vi "test-30frame-QR-static.vi"() -> ()   [LabVIEW 2015]
uses:
  <vilib>/MakerHub/LINX/Public/Peripherals/Digital/Digital Read 1 Chan.vi
  <vilib>/MakerHub/LINX/Public/Peripherals/Digital/Digital Read N Chans.vi
  <vilib>/MakerHub/LINX/Private/Local IO/LinxDigitalRead.vi
  <vilib>/MakerHub/LINX/Public/Utilities/Check Channel.vi
  <vilib>/MakerHub/LINX/Public/Utilities/Open Serial.vi
  <vilib>/MakerHub/LINX/Private/Utilties/Generate Error.vi
  <vilib>/MakerHub/LINX/LMH-LINX.lvlib
  <vilib>/gmath/NI_Gmath.lvlib
panel:
  in  "sensor pin":u8
  in  "Frequency (Hz)":u32=1600
  in  "DIR pin":u8=3
  in  "Pulse pin":u8=4
  out "Form code":bool
  in  "Sensor  Port":refnum<visa-resource-name>="COM3"
  out "data current = data previous ?":bool
  in  "Port Motor":refnum<visa-resource-name>="COM18"
  out "?":T1(plugin-control)
  in  "stop":bool
  out "data-global":string
  out "sum package":dbl
  out "Found?":bool
  out "Mass (kg):":dbl
  out "Tong K/lg (kg)":dbl
  out "Quantity":i32=50
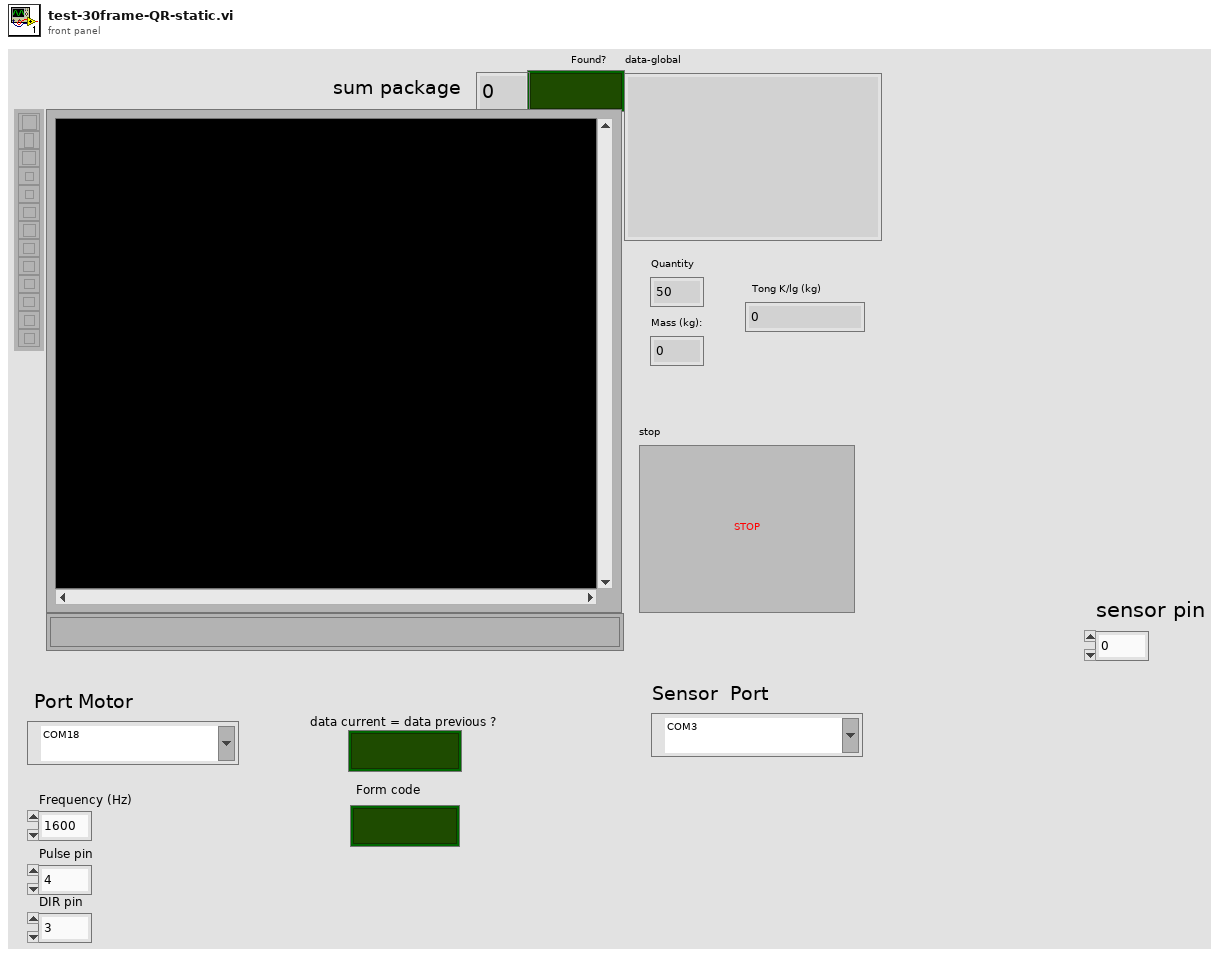
[diagram p1: front panel]
types:
  T1 = typedef "IMAQ Image.ctl" = refnum<image>
  T2 = typedef "LMH-LINX.lvlib/LINX Ref.ctl" = cluster{"IO":T3, "Interface":T4, "LINX Device Config":T5}
  T3 = typedef "LMH-LINX.lvlib/Platform.ctl" = enum16{"Remote", "Local"}
  T4 = typedef "LMH-LINX.lvlib/Interface.ctl" = enum16{"Serial", "TCP"}
  T5 = typedef "LMH-LINX.lvlib/Device.lvlib/LINX Device Config.ctl" = cluster{"Interface":T4, "COM Port":refnum<visa-resource-name>, "TCP Configuration":T6, "Device Family":u8, "Device ID":u8, "Device Name":string, "TCP Ref":refnum<k5>, "Channels":T7}
  T6 = typedef "LMH-LINX.lvlib/Device.lvlib/TCP Config.ctl" = cluster{"IP Address":string, "Port":u16}
  T7 = typedef "LMH-LINX.lvlib/Channels.ctl" = cluster{"DI":u8[], "DO":u8[], "AI":u8[], "AO":u8[], "PWM":u8[], "QE":u8[], "UART":u8[], "I2C 2":u8[], "SPI":u8[], "CAN":u8[], "Servo":u8[], "AI Ref (V)":dbl, "AI Resolution (Bits)":u8, "AO Ref (V)":dbl, "AO Resolution (Bits)":u8}
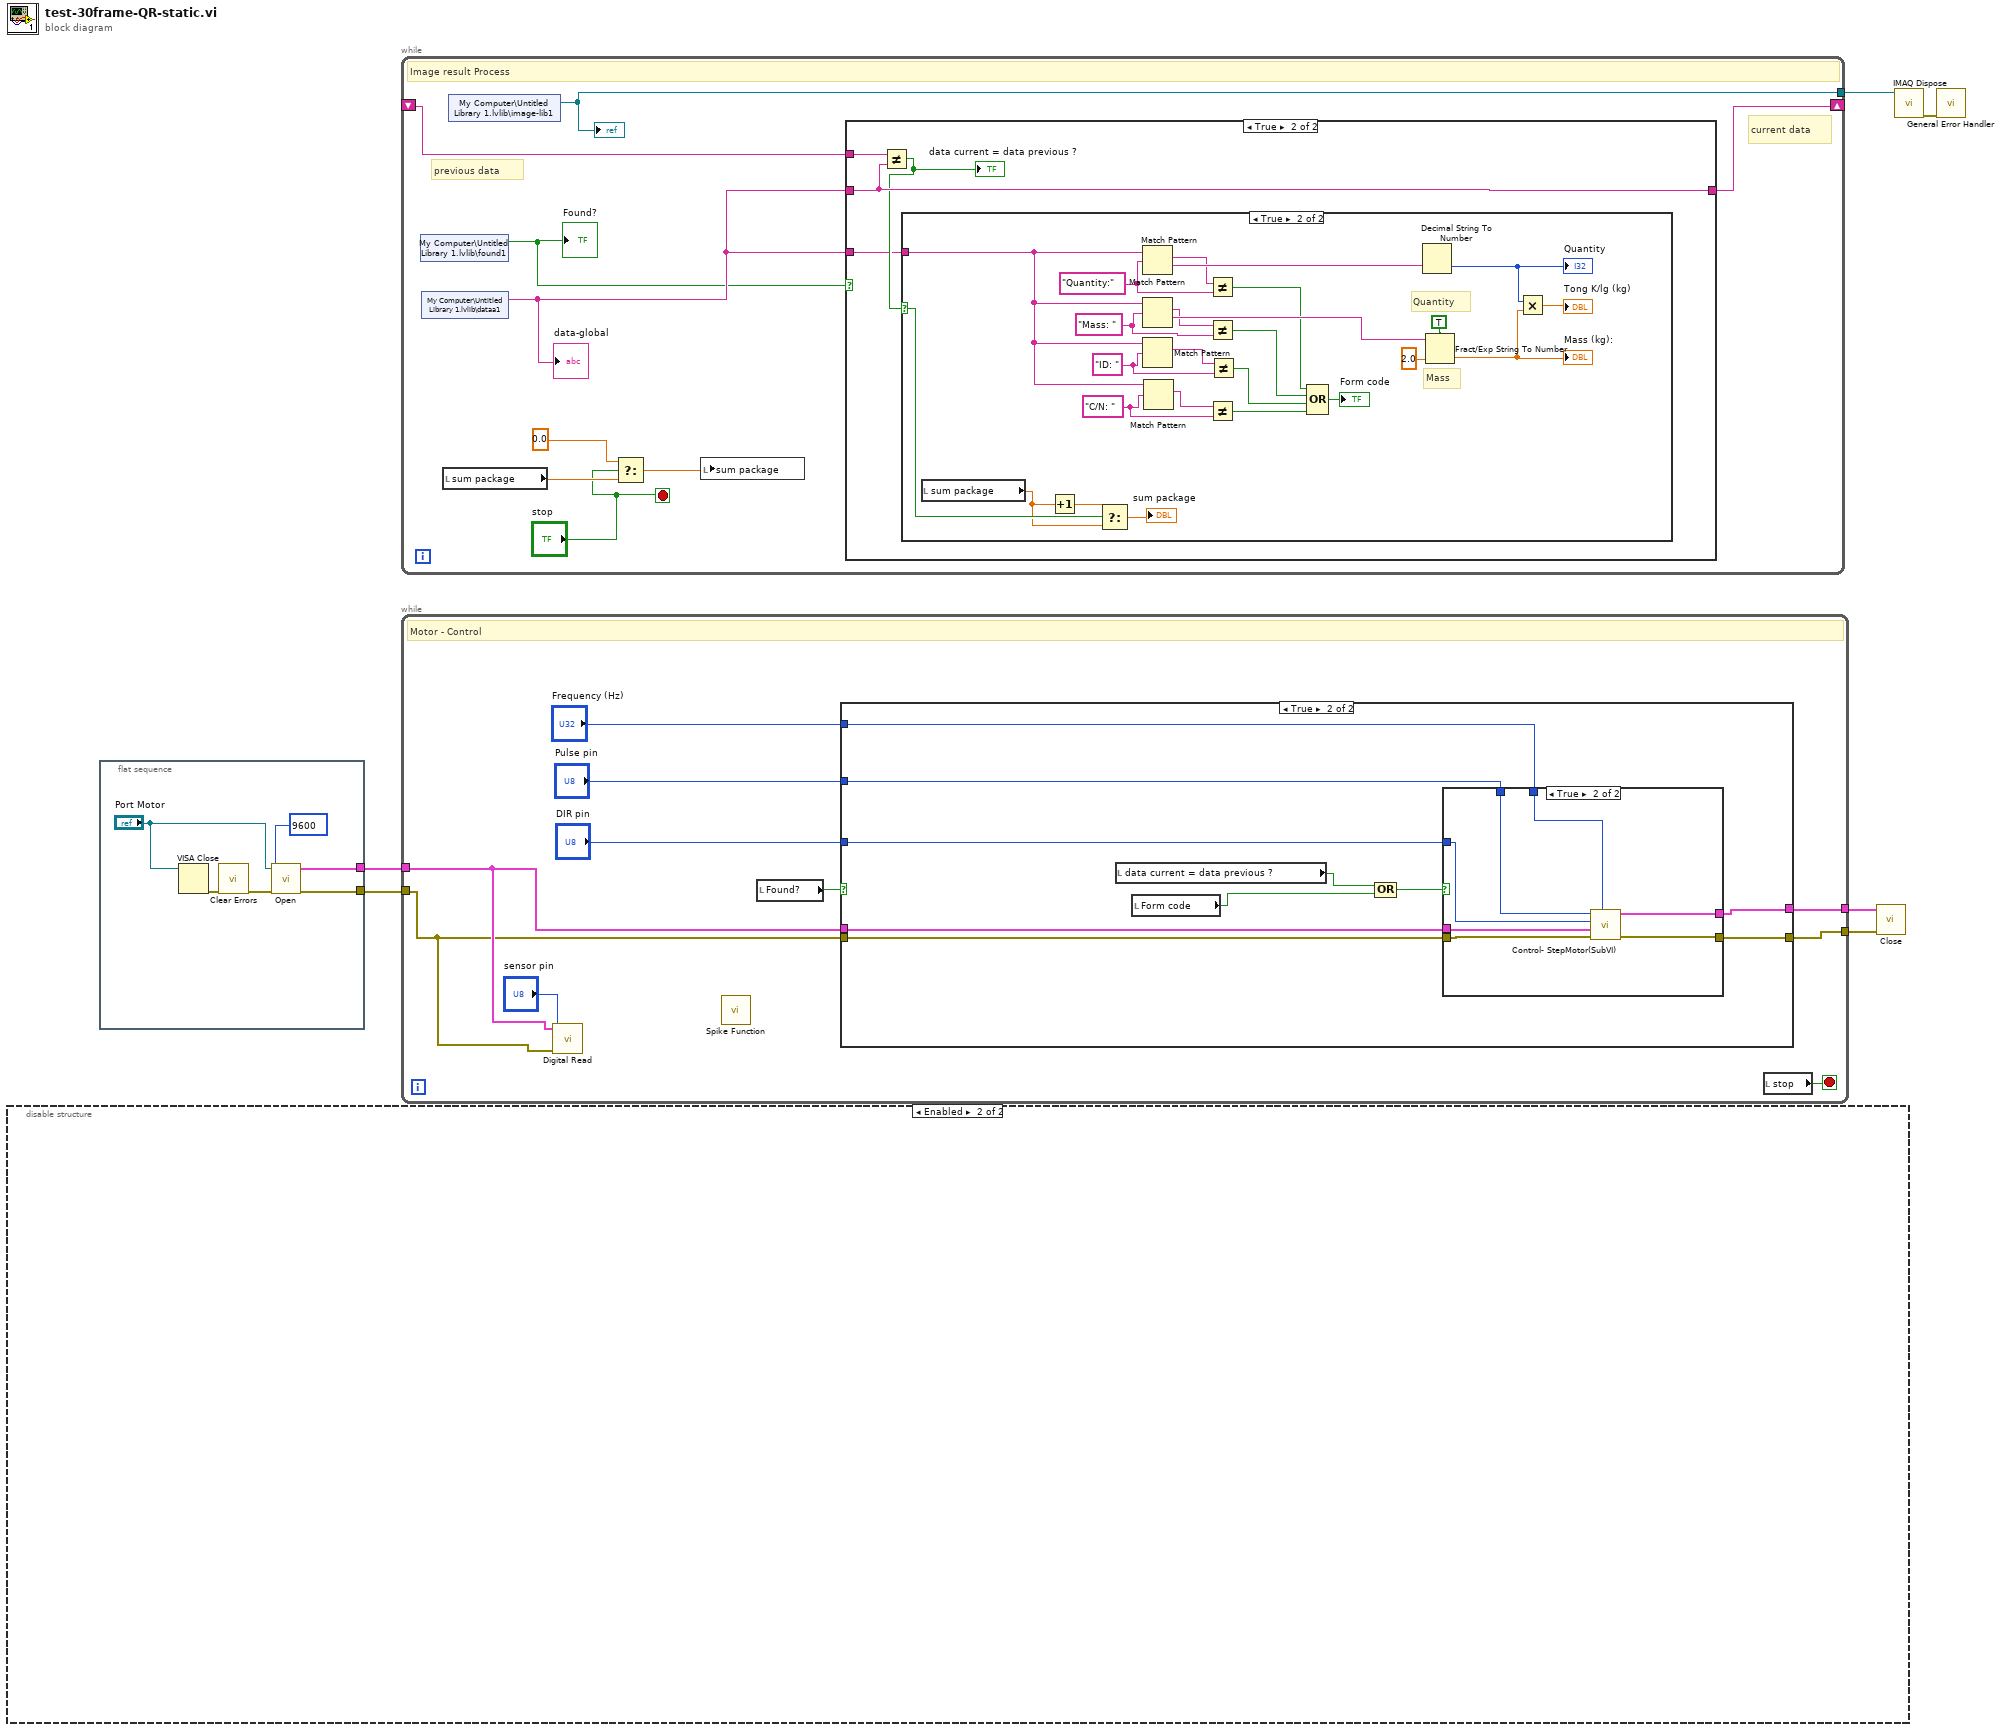
[diagram p0: block diagram]
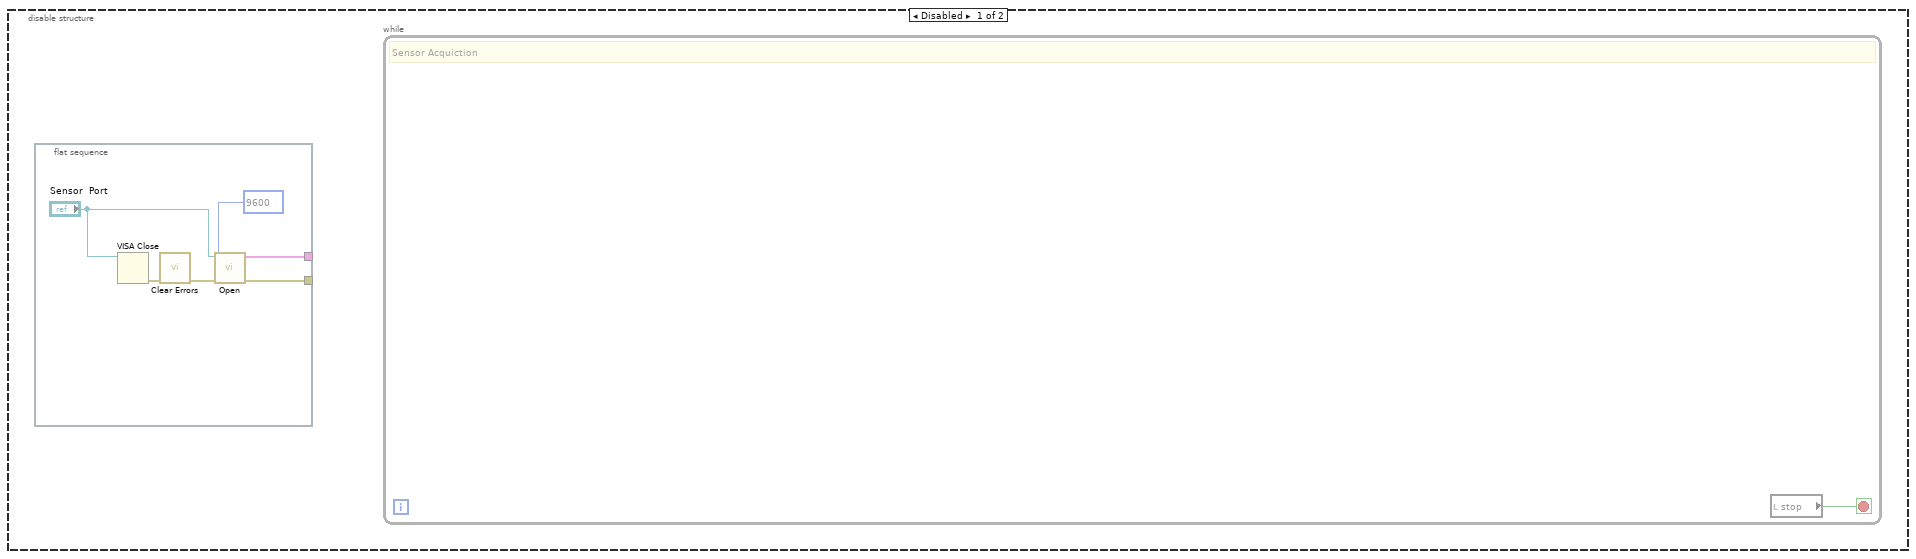
[diagram p2: hidden frame]
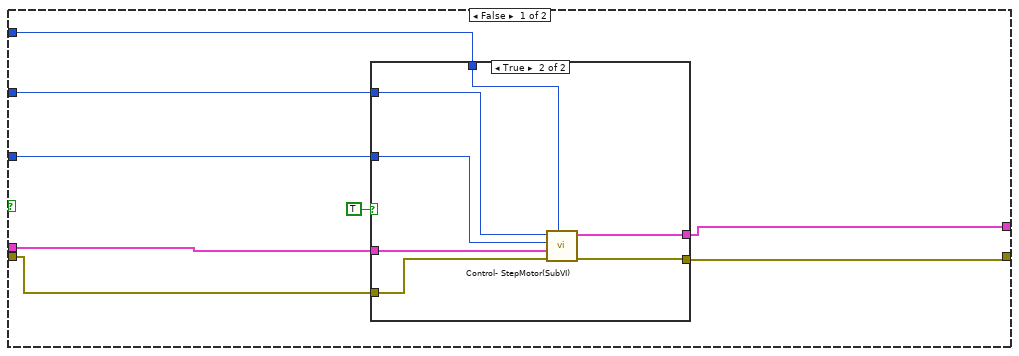
[diagram p3: hidden frame]
diagram:
  n1 = disable-structure shown="Enabled" {
    frame Disabled {
      n2 = flat-sequence {
        tunnel: [w10] -> _
        tunnel: [w9] -> _
        frame #0 {
          n3 = VISA Close(VISA resource name="Sensor  Port") -> (error out=w12:errorcluster)  [unwired: 1 in]
          n4 = call <vilib>:"Clear Errors.vi"("error in (no error)"=w12) -> ("error out"=w11:errorcluster)  [unwired: 5 in, 1 out]
          n5 = call-poly <vilib>:"Open.vi"("Error In"=w11, "Baud Rate Override"=u32 9600, "Serial Port"="Sensor  Port") -> ("Error Out"=w9:errorcluster, "LINX Resource"=w10:T2)  [unwired: 6 in, 1 out]
        }
      }
      n6 = while {
        stop <- w7 stop-if-true
        # "Sensor Acquiction"
        n7 = local read "stop"() -> (w7:bool)
      }
    }
    frame Enabled {
    }
  }
  n8 = flat-sequence {
    tunnel: [w16] -> w4
    tunnel: [w15] -> w3
    frame #0 {
      n9 = VISA Close(VISA resource name="Port Motor") -> (error out=w18:errorcluster)  [unwired: 1 in]
      n10 = call <vilib>:"Clear Errors.vi"("error in (no error)"=w18) -> ("error out"=w17:errorcluster)  [unwired: 5 in, 1 out]
      n11 = call-poly <vilib>:"Open.vi"("Error In"=w17, "Baud Rate Override"=u32 9600, "Serial Port"="Port Motor") -> ("Error Out"=w15:errorcluster, "LINX Resource"=w16:T2)  [unwired: 6 in, 1 out]
    }
  }
  n12 = while {
    shift-right: [w20] -> _
    shift-left: _ -> [w28]
    tunnel: [w21] -> w5
    stop <- "stop" stop-if-true
    # "previous data"
    # "current data"
    # "Image result Process"
    n13 = shared-variable "My Computer\\Untitled Library 1.lvlib\\found1"() -> (w23:bool)  [unwired: 1 in, 1 out]
    "Found?" <- w23
    n14 = shared-variable "My Computer\\Untitled Library 1.lvlib\\dataa1"() -> (w24:string)  [unwired: 1 in, 1 out]
    "data-global" <- w24
    n15 = local read "sum package"() -> (w25:dbl)
    n16 = shared-variable "My Computer\\Untitled Library 1.lvlib\\image-lib1"() -> (w21:refnum<image>)  [unwired: 1 in, 1 out]
    "?" <- w21
    n17 = Select(t=0.0, s="stop", f=w25) -> (s? t:f=w27:dbl)
    n18 = local write "sum package"(w27) -> ()
    n19 = case shown="True" w23 {
      tunnel: w24 -> [_ w30]
      tunnel: [w29 w32] -> w20
      tunnel: w28 -> [w29 w33]
      tunnel: w24 -> [_ w32]
      frame False {
      }
      frame True {
        n20 = Not Equal?(x=w33, y=w32) -> (x != y?=w31:bool)
        "data current = data previous ?" <- w31
        n21 = case shown="True" w31 {
          selector: w31 -> [_ w55]
          tunnel: w30 -> [_ w34]
          frame False {
          }
          frame True {
            w47 = "C/N: " ("regular expression")
            w44 = "ID: " ("regular expression")
            w42 = "Mass: " ("regular expression")
            w40 = "Quantity:" ("regular expression")
            # "Mass"
            # "Quantity"
            n22 = local read "sum package"() -> (w53:dbl)
            n23 = Increment(x=w53) -> (x+1=w54:dbl)
            n24 = Select(t=w54, s=w55, f=w53) -> (s? t:f=→"sum package":dbl)
            n25 = Match Pattern(string=w34, regular expression=w40) -> (match substring=w41:string, after substring=w58:string)  [unwired: 1 in, 2 out]
            n26 = Match Pattern(string=w34, regular expression=w42) -> (match substring=w43:string, after substring=w57:string)  [unwired: 1 in, 2 out]
            n27 = Match Pattern(string=w34, regular expression=w44) -> (match substring=w45:string)  [unwired: 1 in, 3 out]
            n28 = Match Pattern(string=w34, regular expression=w47) -> (match substring=w46:string)  [unwired: 1 in, 3 out]
            n29 = Not Equal?(x=w41, y=w40) -> (x != y?=w39:bool)
            n30 = Not Equal?(x=w43, y=w42) -> (x != y?=w38:bool)
            n31 = Not Equal?(x=w46, y=w47) -> (x != y?=w36:bool)
            n32 = Not Equal?(x=w45, y=w44) -> (x != y?=w37:bool)
            n33 = Compound Arithmetic op=OR(w39, w38, w37, w36) -> (→"Form code":bool)
            n34 = Decimal String To Number(string=w58) -> (number=w51:i32)  [unwired: 2 in, 1 out]
            "Quantity" <- w51
            n35 = Fract/Exp String To Number(use system decimal point (T)=TRUE, string=w57, default (0 dbl)=2.0 ("default (0 DBL)")) -> (number=w49:dbl)  [unwired: 1 in, 1 out]
            "Mass (kg):" <- w49
            n36 = Multiply(x=w51, y=w49) -> (x*y=→"Tong K/lg (kg)":dbl)
          }
        }
      }
    }
  }
  n37 = while {
    tunnel: w4 -> [w61]
    tunnel: w3 -> [w60]
    tunnel: [w67] -> w2
    tunnel: [w63] -> w1
    stop <- w62 stop-if-true
    # "Motor - Control"
    n38 = call-poly <vilib>:"Digital Read.vi"("Error In"=w60, "DI Channel"="sensor pin", "LINX Resource"=w61) -> ()  [unwired: 6 in, 3 out]
    n39 = call <vilib>:"Spike Function.vi"() -> ()  [unwired: 1 in, 1 out]
    n40 = local read "Found?"() -> (w68:bool)
    n41 = case shown="True" w68 {
      tunnel: [w74 w93] -> w67
      tunnel: [w73 w92] -> w63
      tunnel: w61 -> [w76 w90]
      tunnel: w60 -> [w75 w89]
      tunnel: "Frequency (Hz)" -> [w71 w88]
      tunnel: "Pulse pin" -> [w70 w87]
      tunnel: "DIR pin" -> [w69 w86]
      frame False {
        n42 = case shown="True" TRUE {
          tunnel: [w78 w85] -> w74
          tunnel: [w77 w84] -> w73
          tunnel: w76 -> [w78 w83]
          tunnel: w75 -> [w77 w82]
          tunnel: w71 -> [_ w79]
          tunnel: w70 -> [_ w80]
          tunnel: w69 -> [_ w81]
          frame False {
          }
          frame True {
            n43 = call "Control- StepMotor(SubVI).vi"("Frequency (Hz)"=w79, "error in (no error)"=w82, "LINX Resource in"=w83, "DIR pin"=w81, "Pulse pin"=w80) -> ("error out"=w84:errorcluster, "LINX Resource out"=w85:T2)  [unwired: 5 in]
          }
        }
      }
      frame True {
        n44 = local read "data current = data previous ?"() -> (w95:bool)
        n45 = local read "Form code"() -> (w94:bool)
        n46 = Compound Arithmetic op=OR(w95, w94) -> (w91:bool)
        n47 = case shown="True" w91 {
          tunnel: [w97 w104] -> w93
          tunnel: [w96 w103] -> w92
          tunnel: w90 -> [w97 w102]
          tunnel: w89 -> [w96 w101]
          tunnel: w88 -> [_ w100]
          tunnel: w87 -> [_ w99]
          tunnel: w86 -> [_ w98]
          frame False {
          }
          frame True {
            n48 = call "Control- StepMotor(SubVI).vi"("Frequency (Hz)"=w100, "error in (no error)"=w101, "LINX Resource in"=w102, "DIR pin"=w98, "Pulse pin"=w99) -> ("error out"=w103:errorcluster, "LINX Resource out"=w104:T2)  [unwired: 5 in]
          }
        }
      }
    }
    n49 = local read "stop"() -> (w62:bool)
  }
  n50 = call <vilib>:"Close.vi"("Error In"=w1, "LINX Resource"=w2) -> ()  [unwired: 9 in, 1 out]
  n51 = call "IMAQ Dispose"("Image"=w5) -> ("error out"=w6:errorcluster)  [unwired: 5 in]
  n52 = call <vilib>:"General Error Handler.vi"("error in (no error)"=w6) -> ()  [unwired: 10 in, 5 out]
